vi "GPIBsend.vi"(2 "timeout ms":u32=4294967295 format="%.0x", 3 "address string":string, 4 "write buffer":string, 7 "source":string, 8 "write mode (set END:0)":i32, 9 "error in":errorcluster) -> (1 "byte count":i32, 5 "status":bool[](array[boolean]), 6 "error out":errorcluster)   [LabVIEW 2019, in "InstrControl.lvclass"]
doc: "Sends a string to a message based VXI instrument. In order to communicate with an instrument, you must first open the instrument by running the Open VXI Instrument or running the initialize VI (initialize VIs call the Open VXI Instrument in their block diagram). Use the instrument ID generated by the Open VXI Instrument to address the specific instrument, then set the write mode and enter the string to send. If a write error occurs, error code 1230 is returned. If you fail to open the instrument, error code 1232 is returned."
uses:
  InstrControl.lvclass
panel:
  in  "[empty array]":bool[](array[boolean])
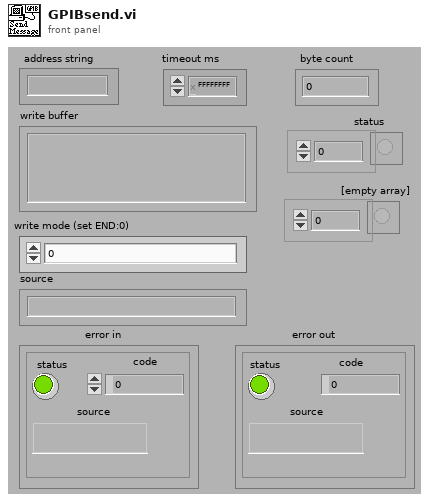
[diagram p1: front panel]
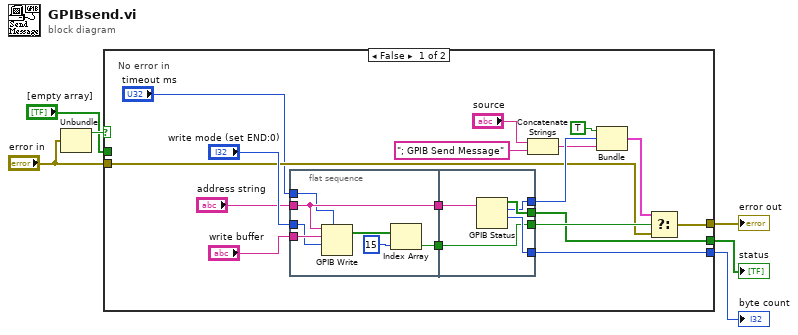
[diagram p0: block diagram]
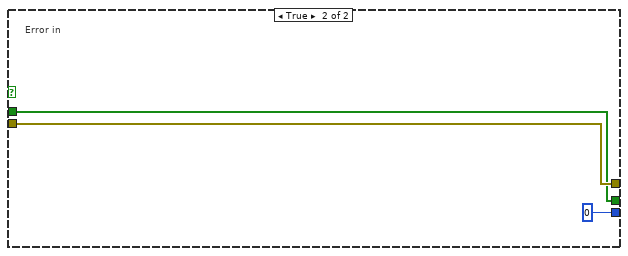
[diagram p2: hidden frame]
diagram:
  n1 = Unbundle("error in") -> ("status"=w2:bool)  [unwired: 2 out]
  n2 = case shown="False" w2 {
    tunnel: "[empty array]" -> [_ w36]
    tunnel: [w16 w36] -> w3
    tunnel: [w22 w37] -> w4
    tunnel: "error in" -> [w12 w37]
    tunnel: [w17 0] -> w6
    frame False {
      # "No error in"
      n3 = flat-sequence {
        tunnel: [w27] -> w8
        tunnel: "write mode (set END:0)" -> [w24]
        tunnel: "write buffer" -> [w28]
        tunnel: "address string" -> [w26]
        tunnel: [w26] -> w7
        tunnel: "timeout ms" -> [w25]
        tunnel: [w34] -> w16
        tunnel: [w35] -> w17
        tunnel: [w31] -> w18
        tunnel: w8 -> [w31]
        tunnel: [w33] -> w15
        tunnel: w7 -> [w32]
        frame #0 {
          n4 = GPIB Write(0:w26, 1:w28, 2:w24, 4:w25) -> (5:w29:bool[])  [unwired: 1 in, 1 out]
          n5 = Index Array(array=w29, index=15) -> (element=w27:bool)
        }
        frame #1 {
          n6 = GPIB Status(0:w32) -> (2:w34:bool[], 3:w33:i16, 4:w35:i32)  [unwired: 1 in, 1 out]
        }
      }
      n7 = Concatenate Strings("source", "; GPIB Send Message") -> (w13:string)
      n8 = Bundle(TRUE, "GPIB error"=w15, w13) -> (w23:cluster{bool, "GPIB error":i16, string})  [unwired: 1 in]
      n9 = Select(t=w23, s=w18, f=w12) -> (s? t:f=w22:errorcluster)
    }
    frame True {
      # "Error in"
    }
  }
  "status" <- w3
  "error out" <- w4
  "byte count" <- w6
